vi "SUB_WR_COM1_CbyCFindString_timeout_way2.vi"(4 "Begin time":dbl, 5 "Find this String":string, 6 "Timeout Seccond":dbl, 7 "cmd string":string, 8 "duplicate VISA resource name 2":refnum<visa-resource-name>) -> (0 "VISA out":refnum<visa-resource-name>, 1 "Output String":string, 2 "spent seconds":dbl, 3 "Found String":bool)   [LabVIEW 2011]
panel:
  out "String":string
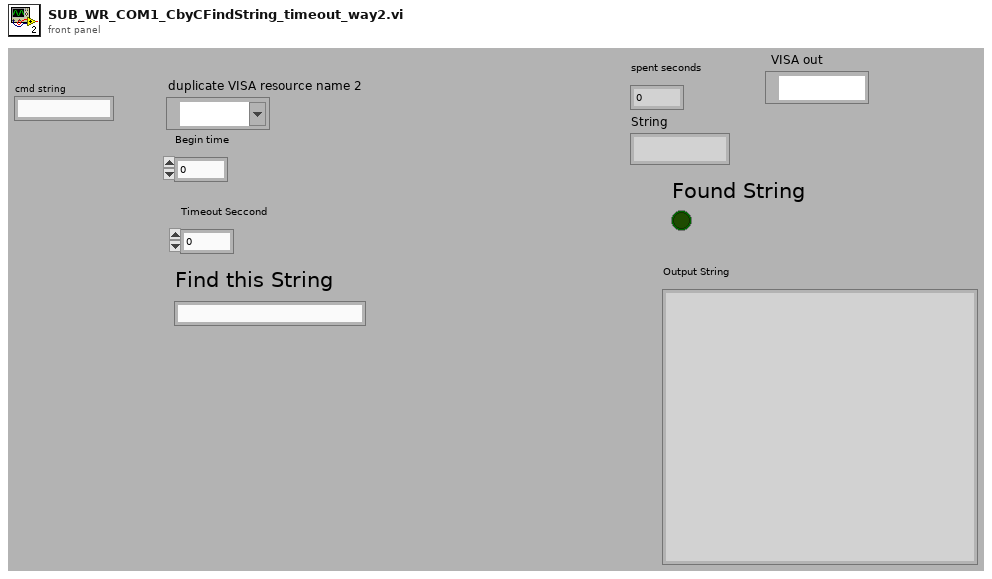
[diagram p1: front panel]
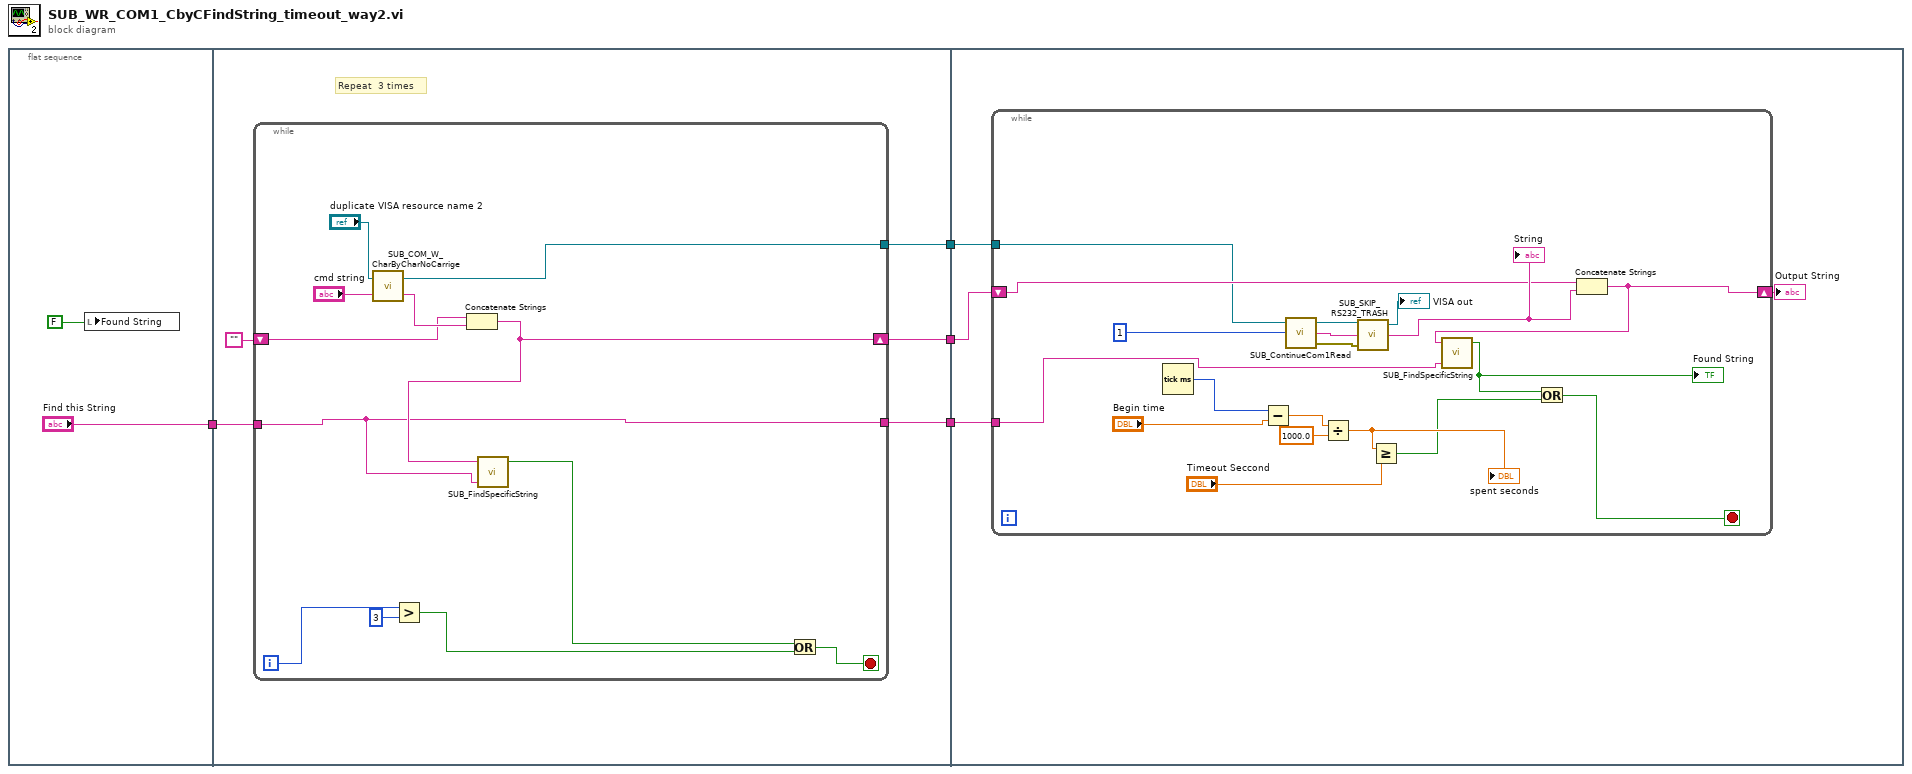
[diagram p0: block diagram]
diagram:
  n1 = flat-sequence {
    tunnel: ["Find this String"] -> w2
    tunnel: [w10] -> w4
    tunnel: [w9] -> w3
    tunnel: w2 -> [w8]
    tunnel: [w7] -> w1
    tunnel: w4 -> [w26]
    tunnel: w3 -> [w25]
    tunnel: w1 -> [w24]
    frame #0 {
      n2 = local write "Found String"(FALSE) -> ()
    }
    frame #1 {
      # "Repeat  3 times"
      n3 = while {
        shift-right: [w19] -> w10
        shift-left: "" -> [w21]
        tunnel: [w20] -> w9
        tunnel: [w18] -> w7
        tunnel: w8 -> [w18]
        i -> [w17]
        stop <- w15 stop-if-true
        n4 = call "SUB_COM_W_CharByCharNoCarrige.vi"("cmd string"="cmd string", "duplicate VISA resource name"="duplicate VISA resource name 2") -> ("OUT string"=w22:string, "VISA resource OUT"=w20:refnum<visa-resource-name>)
        n5 = Greater?(x=w17, y=3) -> (0:w16:bool)
        n6 = Concatenate Strings(w21, w22) -> (w19:string)
        n7 = call "SUB_FindSpecificString.vi"("Find this String"=w18, "String data"=w19) -> ("Found"=w13:bool)  [unwired: 2 in, 1 out]
        n8 = Or(x=w13, y=w16) -> (x .or. y?=w15:bool)
      }
    }
    frame #2 {
      n9 = while {
        shift-right: [w30] -> w27
        shift-left: w26 -> [w34]
        tunnel: w25 -> [w28]
        tunnel: w24 -> [w29]
        stop <- w36 stop-if-true
        n10 = Tick Count (ms)() -> (millisecond timer value=w33:u32)
        n11 = Subtract(x=w33, y="Begin time") -> (x-y=w42:dbl)
        n12 = call "SUB_ContinueCom1Read.vi"("Numeric"=1, "duplicate VISA resource name 2"=w28) -> ("error out"=w44:errorcluster, "String"=w45:string, "duplicate VISA resource name"=w46:refnum<visa-resource-name>)  [unwired: 1 in]
        n13 = Divide(x=w42, y=1000.0) -> (x/y=w40:dbl)
        "spent seconds" <- w40
        n14 = call "SUB_SKIP_RS232_TRASH.vi"("error out 2"=w44, "read buffer"=w45, "duplicate VISA resource name 2"=w46) -> ("String"=w35:string, "duplicate VISA resource name"=→"VISA out":refnum<visa-resource-name>)  [unwired: 1 out]
        "String" <- w35
        n15 = Greater Or Equal?(x=w40, y="Timeout Seccond") -> (x >= y?=w37:bool)
        n16 = Concatenate Strings(w34, w35) -> (w30:string)
        n17 = call "SUB_FindSpecificString.vi"("Find this String"=w29, "String data"=w30) -> ("Found"=w38:bool)  [unwired: 2 in, 1 out]
        "Found String" <- w38
        n18 = Or(x=w38, y=w37) -> (x .or. y?=w36:bool)
      }
      "Output String" <- w27
    }
  }
